vi "Remove Off Field Items.vi"(10 "Field":T1, 11 "JSONCluster in":T2) -> (3 "JSONCluster out":T2)   [LabVIEW 2015]
uses:
  Typedef/JSONCluster.ctl
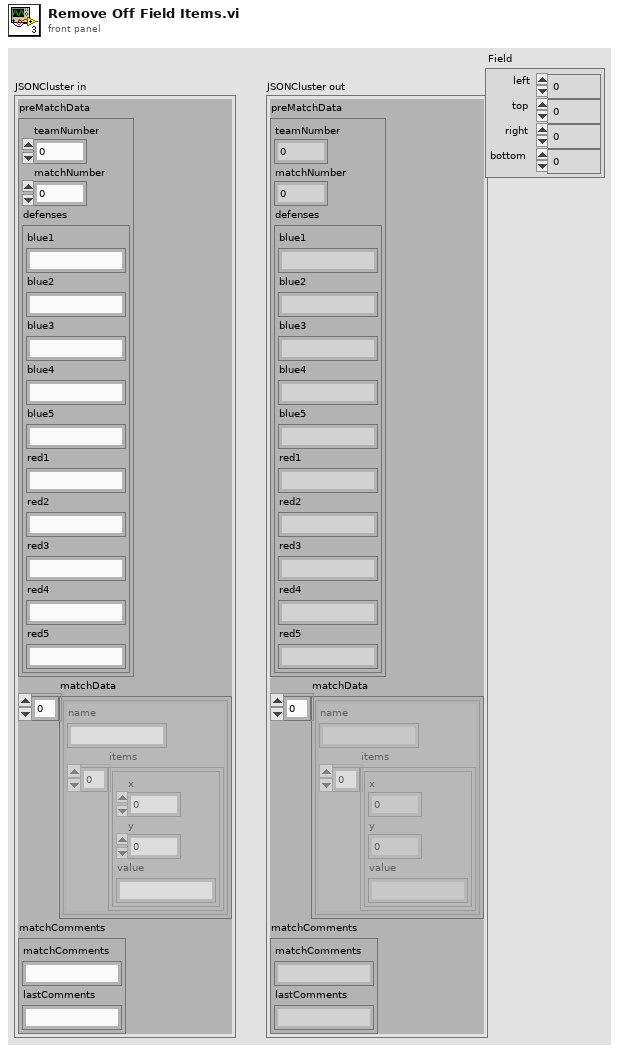
[diagram p1: front panel]
types:
  T1 = cluster{"left":i16, "top":i16, "right":i16, "bottom":i16}
  T2 = typedef "JSONCluster.ctl" = cluster{"preMatchData":cluster{"teamNumber":i32, "matchNumber":i32, "defenses":cluster{"blue1":string, "blue2":string, "blue3":string, "blue4":string, "blue5":string, "red1":string, "red2":string, "red3":string, "red4":string, "red5":string}}, "matchData":cluster{"name":string, "items":cluster{"x":i32, "y":i32, "value":string}[]}[], "matchComments":cluster{"matchComments":string, "lastComments":string}}
  T3 = cluster{"name":string, "items":cluster{"x":i32, "y":i32, "value":string}[]}[]
  T4 = cluster{"name":string, "items":cluster{"x":i32, "y":i32, "value":string}[]}
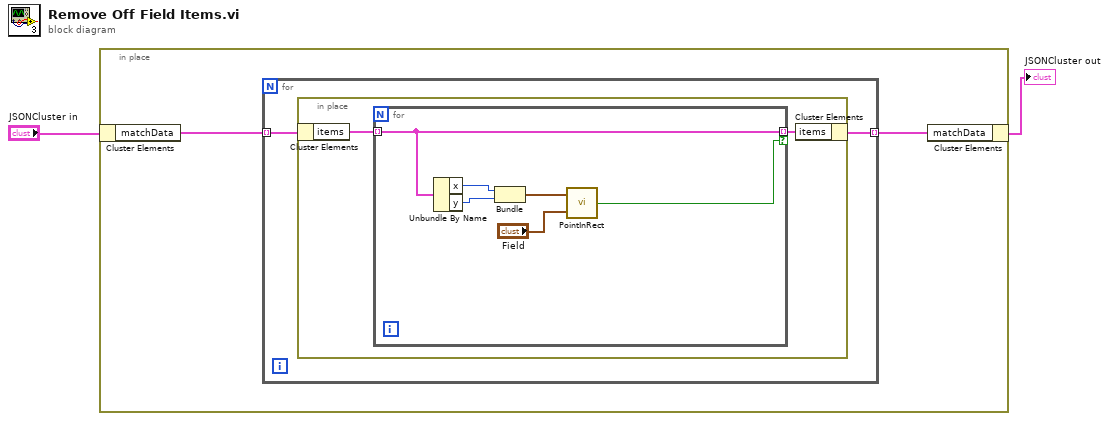
[diagram p0: block diagram]
diagram:
  n1 = in-place {
    n2 = in-place-cluster #1("JSONCluster in") -> ("matchData"=w4:T3)
    n3 = for {
      tunnel: w4 -> [w6] mode=indexing
      tunnel: [w5] -> w3 mode=indexing
      n4 = in-place {
        n5 = in-place-cluster #2(w6) -> ("items"=w8:cluster{"x":i32, "y":i32, "value":string}[])
        n6 = for {
          tunnel: w8 -> [w14] mode=indexing
          tunnel: [w14] -> w7 mode=indexing if=w9
          n7 = Unbundle By Name(w14) -> ("x"=w13:i32, "y"=w12:i32)
          n8 = Bundle("x"=w13, "y"=w12) -> (w11:cluster{"x":i32, "y":i32})  [unwired: 1 in]
          n9 = call <vilib>:"PointInRect.vi"("rect"="Field", "point"=w11) -> ("pt in rect"=w9:bool)
        }
        n10 = in-place-cluster #2("items"=w7) -> (w5:T4)
      }
    }
    n11 = in-place-cluster #1("matchData"=w3) -> (→"JSONCluster out":T2)
  }
